vi "komutator.vi"() -> ()   [LabVIEW 2016]
uses:
  <userlib>/Open_device_2015.llb/Select_Instr.ctl
panel:
  out "error out":errorcluster
  in  "Select_Instrument":T1="TCPIP::156.17.45.35::inst23::INSTR"
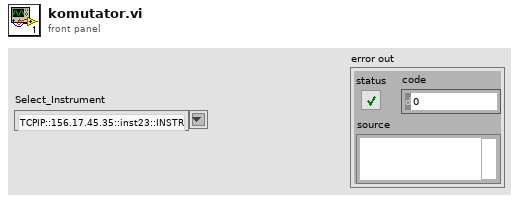
[diagram p1: front panel]
types:
  T1 = typedef "Select_Instr.ctl" = string
  T2 = cluster{"VISA resource name":refnum<visa-resource-name>}
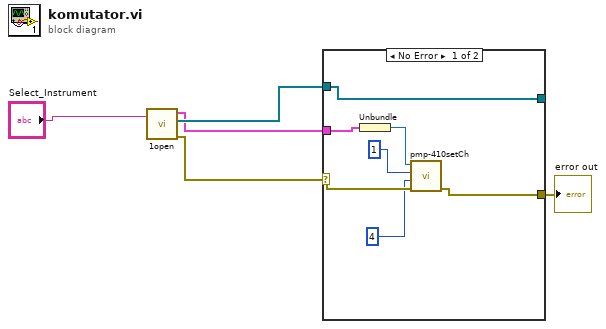
[diagram p0: block diagram]
diagram:
  n1 = call <userlib>:"1open.vi"("VISA resource name"="Select_Instrument") -> ("InstrCluster"=w1:T2, "InstrArray"=w2:refnum<visa-resource-name>[], "error out"=w4:errorcluster)  [unwired: 1 in, 1 out]
  n2 = case shown="No Error" w4 {
    selector: w4 -> [w12 w13]
    tunnel: [w11 w13] -> w3
    tunnel: w2 -> [w10 w14]
    tunnel: [w10 w14] -> _
    tunnel: w1 -> [w9 _]
    frame No Error {
      n3 = Unbundle(w9) -> ("VISA resource name"=w8:refnum<visa-resource-name>)
      n4 = call <userlib>:"pmp-410setCh.vi"("error in (no error)"=w12, "Channel"=4, "Slave#"=1, "VISA Refnum in"=w8) -> ("error out"=w11:errorcluster)  [unwired: 6 in, 1 out]
    }
    frame Error {
    }
  }
  "error out" <- w3
